vi "PID Advanced.vi"(6 "reinitialize? (F)":bool, 7 "output range":cluster{"output high":dbl, "output low":dbl}={"output high"=100.0, "output low"=-100.0} {"output low" format="%.2f"; "output high" format="%.2f"}, 8 "dt (s)":dbl=-1.0 format="%.3f", 9 "PID gains":T1={"proportional gain (Kc)"=1.0, "integral time (Ti, min)"=0.01, "derivative time (Td, min)"=0.0} {"derivative time (Td, min)" format="%.3f"; "integral time (Ti, min)" format="%.3f"; "proportional gain (Kc)" format="%.3f"}, 10 "process variable":dbl step=0.01 format="%.2f", 11 "setpoint":dbl step=0.01 format="%.2f") -> (0 "dt out (s)":dbl format="%.3f", 3 "output":dbl format="%.2f")   [LabVIEW 2019, in "control.lvlib"]
uses:
  control.lvlib
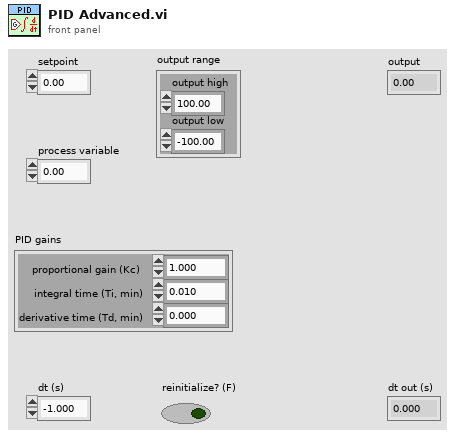
[diagram p1: front panel]
types:
  T1 = cluster{"proportional gain (Kc)":dbl, "integral time (Ti, min)":dbl, "derivative time (Td, min)":dbl}
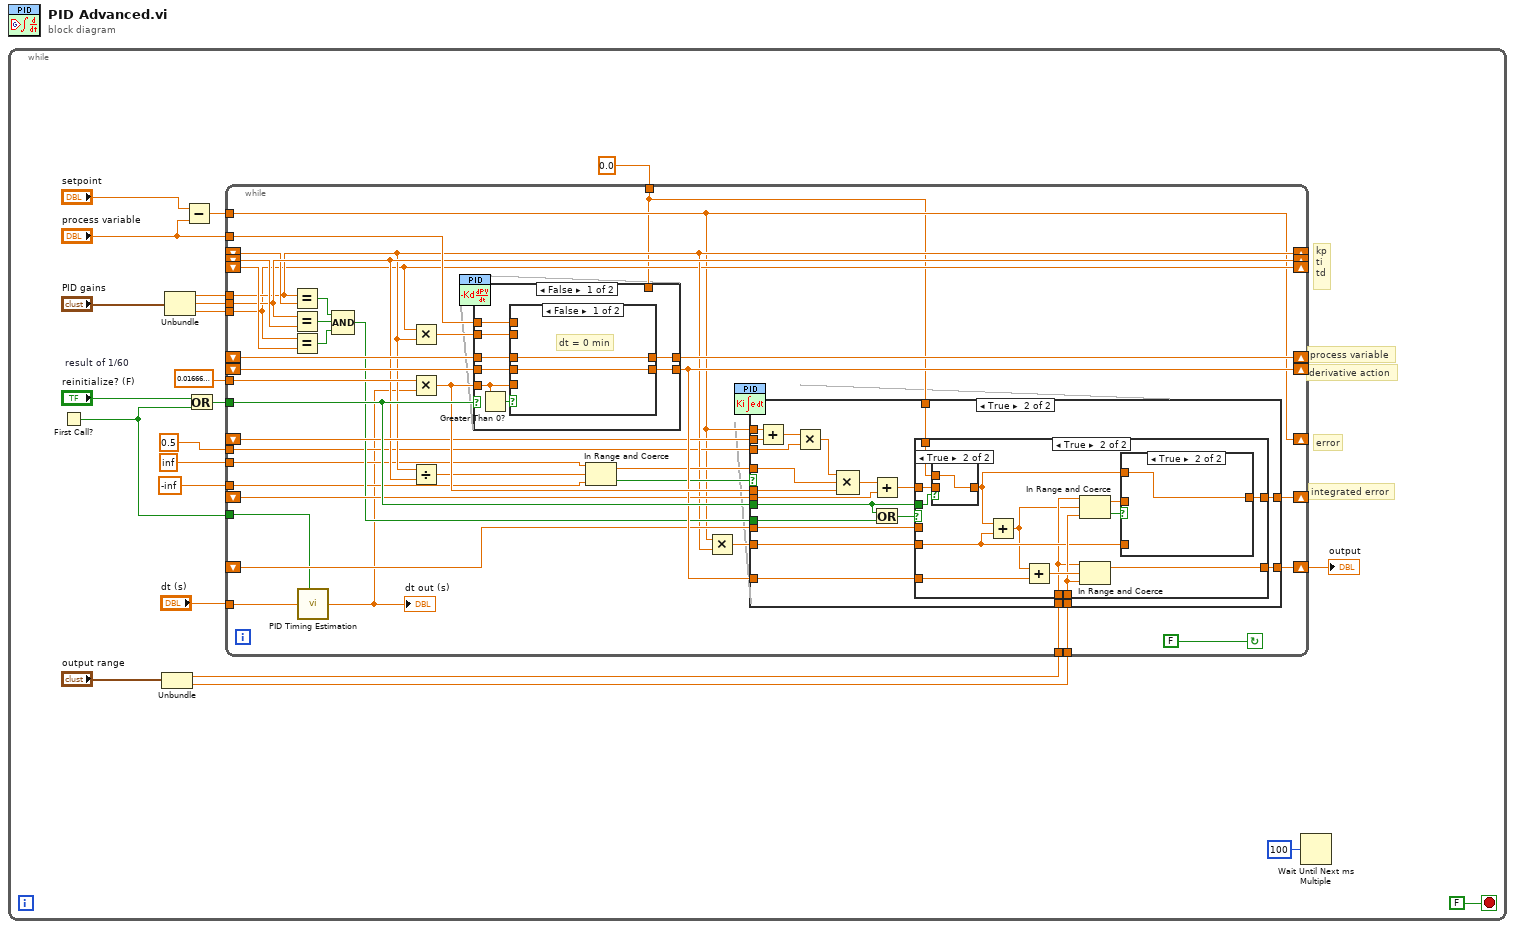
[diagram p0: block diagram]
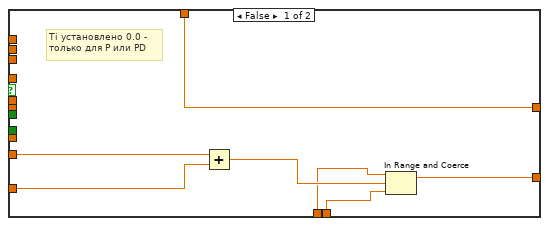
[diagram p2: hidden frame]
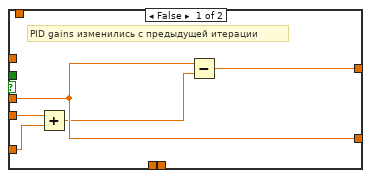
[diagram p3: hidden frame]
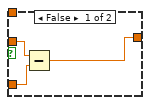
[diagram p4: hidden frame]
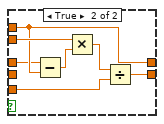
[diagram p6: hidden frame]
diagram:
  n1 = while {
    stop <- FALSE stop-if-true
    w7 = 0.016666666666666666  # result of 1/60
    # "derivative action"
    # "process variable"
    # "kp\nti\ntd"
    # "error"
    # "integrated error"
    n2 = First Call?() -> (First Call?: T/F=w20:bool)
    n3 = Unbundle("output range") -> ("output high"=w5:dbl, "output low"=w6:dbl)
    n4 = Unbundle("PID gains") -> ("proportional gain (Kc)"=w2:dbl, "integral time (Ti, min)"=w3:dbl, "derivative time (Td, min)"=w4:dbl)
    n5 = Subtract(x="setpoint", y="process variable") -> (x-y=w18:dbl)
    n6 = Or(x="reinitialize? (F)", y=w20) -> (x .or. y?=w1:bool)
    n7 = while {
      tunnel: w1 -> [w61]
      shift-right: [w33] -> _
      shift-left: _ -> [w34]
      shift-right: [w35] -> _
      shift-left: _ -> [w58]
      shift-right: [w28] -> _
      shift-left: _ -> [w59]
      tunnel: w2 -> [w33]
      tunnel: w3 -> [w35]
      tunnel: w4 -> [w28]
      tunnel: "dt (s)" -> [w24]
      tunnel: w5 -> [w54]
      tunnel: w6 -> [w53]
      tunnel: "process variable" -> [w52]
      shift-right: [w51] -> _
      shift-left: _ -> [w50]
      shift-right: [w49] -> _
      shift-left: _ -> [w41]
      shift-right: [w48] -> w14
      shift-left: _ -> [w47]
      shift-right: [w27] -> _
      shift-left: _ -> [w46]
      shift-right: [w45] -> _
      shift-left: _ -> [w44]
      tunnel: w7 -> [w38]
      tunnel: 0.5 ("y") -> [w32]
      tunnel: inf ("upper limit") -> [w30]
      tunnel: -inf ("lower limit") -> [w31]
      tunnel: w18 -> [w27]
      tunnel: 0.0 -> [w26]
      tunnel: w20 -> [w25]
      stop <- FALSE continue-if-true
      n8 = Equal?(x=w33, y=w34) -> (x = y?=w56:bool)
      n9 = Equal?(x=w35, y=w58) -> (x = y?=w55:bool)
      n10 = Equal?(x=w28, y=w59) -> (x = y?=w57:bool)
      n11 = call "PID Timing Estimation.vi"("R"=w25, "dt (s) in"=w24) -> ("dt (s) out"=w23:dbl)  [unwired: 7 in]
      "dt out (s)" <- w23
      n12 = Compound Arithmetic op=AND(w56, w55, w57) -> (w36:bool)
      n13 = Multiply(x=w28, y=w33) -> (x*y=w40:dbl)
      n14 = Multiply(x=w38, y=w23) -> (x*y=w60:dbl)
      n15 = Divide(x=w33, y=w35) -> (x/y=w39:dbl)
      n16 = case shown="False" w61 {
        tunnel: w50 -> [w122 _]
        tunnel: w40 -> [w119 _]
        tunnel: w52 -> [w121 w133]
        tunnel: [w118 w133] -> w51
        tunnel: [w120 w132] -> w49
        tunnel: w41 -> [w116 _]
        tunnel: w60 -> [w115 _]
        tunnel: w26 -> [_ w132]
        frame False {
          n17 = Greater Than 0?(x=w115) -> (x > 0?=w117:bool)
          n18 = case shown="False" w117 {
            tunnel: w122 -> [w124 w125]
            tunnel: w115 -> [_ w130]
            tunnel: w121 -> [_ w126]
            tunnel: [w123 w129] -> w120
            tunnel: w119 -> [_ w128]
            tunnel: [w124 w126] -> w118
            tunnel: w116 -> [w123 _]
            frame False {
              # "dt = 0 min"
            }
            frame True {
              n19 = Subtract(x=w125, y=w126) -> (x-y=w127:dbl)
              n20 = Multiply(x=w128, y=w127) -> (x*y=w131:dbl)
              n21 = Divide(x=w131, y=w130) -> (x/y=w129:dbl)
            }
          }
        }
        frame True {
        }
      }
      n22 = In Range and Coerce(upper limit=w30, x=w39, lower limit=w31) -> (coerced(x)=w43:dbl, In Range?=w42:bool)
      n23 = Multiply(x=w27, y=w33) -> (x*y=w37:dbl)
      n24 = case shown="True" w42 {
        tunnel: w27 -> [_ w88]
        tunnel: w46 -> [_ w89]
        tunnel: w44 -> [_ w84]
        tunnel: [w62 w79] -> w45
        tunnel: w43 -> [_ w77]
        tunnel: w37 -> [w67 w82]
        tunnel: [w68 w78] -> w48
        tunnel: w47 -> [_ w80]
        tunnel: w49 -> [w66 w76]
        tunnel: w61 -> [_ w75]
        tunnel: w36 -> [_ w74]
        tunnel: w60 -> [_ w73]
        tunnel: w54 -> [w64 w71]
        tunnel: w53 -> [w63 w72]
        tunnel: w32 -> [_ w70]
        tunnel: w26 -> [w62 w69]
        frame False {
          # "Ti установлено 0.0 -\nтолько для P или PD"
          n25 = Add(x=w67, y=w66) -> (x+y=w65:dbl)
          n26 = In Range and Coerce(upper limit=w64, x=w65, lower limit=w63) -> (coerced(x)=w68:dbl)  [unwired: 1 out]
        }
        frame True {
          n27 = Add(x=w88, y=w89) -> (x+y=w87:dbl)
          n28 = Multiply(x=w87, y=w70) -> (x*y=w86:dbl)
          n29 = Compound Arithmetic op=MULTIPLY(w86, w77, w73) -> (w85:dbl)
          n30 = Add(x=w85, y=w84) -> (x+y=w83:dbl)
          n31 = Or(x=w75, y=w74) -> (x .or. y?=w81:bool)
          n32 = case shown="True" w81 {
            tunnel: w83 -> [_ w102]
            tunnel: w82 -> [w92 w97]
            tunnel: w80 -> [w94 _]
            tunnel: w75 -> [_ w104]
            tunnel: [w93 w99] -> w79
            tunnel: [w94 w107] -> w78
            tunnel: w76 -> [w91 w106]
            tunnel: w72 -> [_ w105]
            tunnel: w71 -> [_ w96]
            tunnel: w69 -> [_ w103]
            frame False {
              # "PID gains изменились с предыдущей итерации"
              n33 = Add(x=w92, y=w91) -> (x+y=w90:dbl)
              n34 = Subtract(x=w94, y=w90) -> (x-y=w93:dbl)
            }
            frame True {
              n35 = case shown="True" w104 {
                tunnel: w103 -> [_ w114]
                tunnel: [w113 w114] -> w101
                tunnel: w102 -> [w113 _]
                frame False {
                }
                frame True {
                }
              }
              n36 = Add(x=w101, y=w97) -> (x+y=w95:dbl)
              n37 = Add(x=w95, y=w106) -> (x+y=w108:dbl)
              n38 = In Range and Coerce(upper limit=w96, x=w95, lower limit=w105) -> (coerced(x)=w98:dbl, In Range?=w100:bool)
              n39 = In Range and Coerce(upper limit=w96, x=w108, lower limit=w105) -> (coerced(x)=w107:dbl)  [unwired: 1 out]
              n40 = case shown="True" w100 {
                tunnel: w101 -> [_ w112]
                tunnel: [w109 w112] -> w99
                tunnel: w98 -> [w111 _]
                tunnel: w97 -> [w110 _]
                frame False {
                  n41 = Subtract(x=w111, y=w110) -> (x-y=w109:dbl)
                }
                frame True {
                }
              }
            }
          }
        }
      }
    }
    "output" <- w14
    n42 = Wait Until Next ms Multiple(millisecond multiple=u32 100) -> ()  [unwired: 1 out]
  }
